vi "Get RM_RI (SubVI).vi"(10 "Bwd":dbl[](array[numeric]), 11 "Fwd":dbl[](array[numeric])) -> (3 "Reflection Markers":T1)   [LabVIEW 2017]
panel:
  in  "Flow Rate (ml/s)":waveform(dbl)
  in  "Pressure (mmHg)":waveform(dbl)
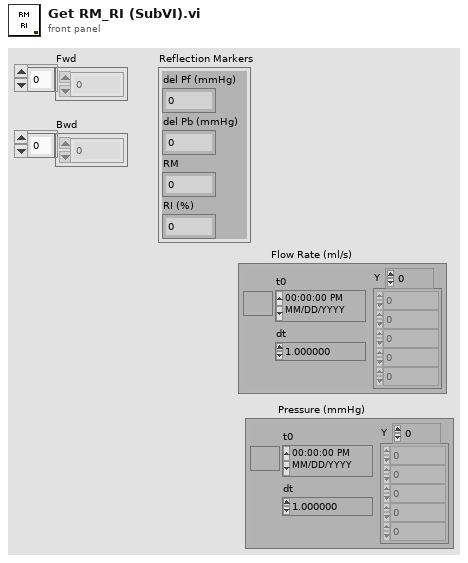
[diagram p1: front panel]
types:
  T1 = cluster{"del Pf (mmHg)":dbl, "del Pb (mmHg)":dbl, "RM":dbl, "RI (%)":dbl}
  T2 = cluster{"del Pf":dbl, "del Pb":dbl, "RM":dbl, "RI (%)":dbl}
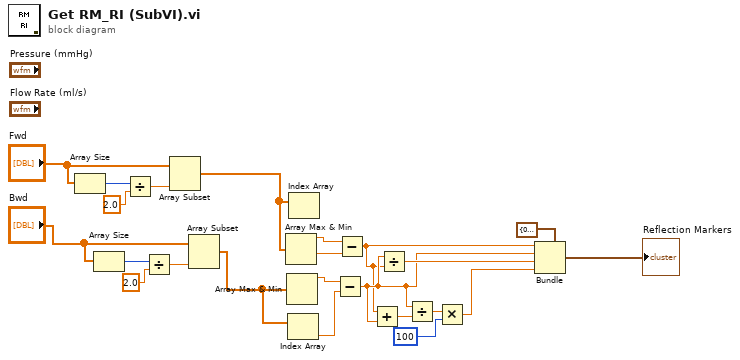
[diagram p0: block diagram]
diagram:
  n1 = Array Size(array="Fwd") -> (size(s)=w11:i32)
  n2 = Array Size(array="Bwd") -> (size(s)=w7:i32)
  n3 = Divide(x=w11, y=2.0 ("Min Value")) -> (x/y=w10:dbl)
  n4 = Divide(x=w7, y=2.0 ("Min Value")) -> (x/y=w6:dbl)
  n5 = Array Subset(array="Fwd", length=w10) -> (w4:dbl[])  [unwired: 1 in]
  n6 = Array Subset(array="Bwd", length=w6) -> (w3:dbl[])  [unwired: 1 in]
  n7 = Array Max & Min(array=w4) -> (max value=w14:dbl, min value=w2:dbl)  [unwired: 2 out]
  n8 = Array Max & Min(array=w3) -> (max value=w13:dbl)  [unwired: 3 out]
  n9 = Index Array(array=w3) -> (element=w1:dbl)  [unwired: 1 in]
  n10 = Index Array(array=w4) -> ()  [unwired: 1 in, 1 out]
  n11 = Subtract(x=w13, y=w1) -> (x-y=w19:dbl)
  n12 = Subtract(x=w14, y=w2) -> (x-y=w18:dbl)
  n13 = Add(x=w18, y=w19) -> (x+y=w15:dbl)
  n14 = Divide(x=w19, y=w18) -> (x/y=w20:dbl)
  n15 = Divide(x=w19, y=w15) -> (x/y=w16:dbl)
  n16 = Multiply(x=w16, y=100) -> (x*y=w21:dbl)
  n17 = Bundle(cluster=T2 {"del Pf"=0.0, "del Pb"=0.0, "RM"=0.0, "RI (%)"=0.0}, "del Pf"=w18, "del Pb"=w19, "RM"=w20, "RI (%)"=w21) -> (→"Reflection Markers":T2)
